vi "read max #frames.vi"(8 "error in (no error)":errorcluster, 11 "Simulated_CCD_Camera in":refnum<class "Sim_CCD.lvclass">) -> (0 "error out":errorcluster, 2 "max #pix":i64[][](array[numeric]), 3 "Simulated_CCD_Camera out":refnum<class "Sim_CCD.lvclass">)   [LabVIEW 2018, in "Sim_CCD.lvclass"]
uses:
  Sim_CCD.lvclass
  Sim_CCD.lvclass/Sim_CCD.ctl
  <vilib>/Utility/file.llb/Read Delimited Spreadsheet (I64).vi
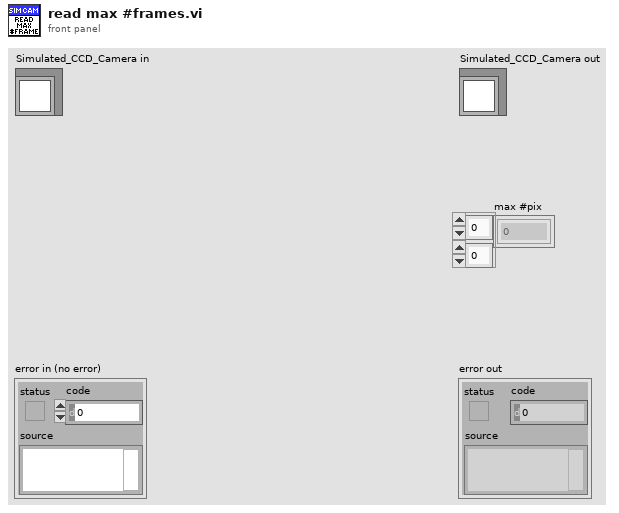
[diagram p1: front panel]
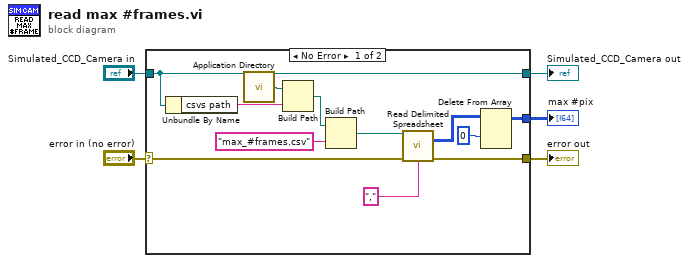
[diagram p0: block diagram]
diagram:
  n1 = case shown="No Error" "error in (no error)" {
    selector: "error in (no error)" -> [w16 w19]
    tunnel: [w15 w19] -> w4
    tunnel: [w14 w18] -> w2
    tunnel: "Simulated_CCD_Camera in" -> [w14 w18]
    tunnel: [w7 _] -> w1
    frame No Error {
      n2 = Unbundle By Name(w14) -> ("csvs path"=w9:string)
      n3 = call <vilib>:"Application Directory.vi"() -> ("Application Directory"=w13:path)
      n4 = Build Path(base path=w13, name or relative path=w9) -> (appended path=w12:path)
      n5 = Build Path(base path=w12, name or relative path="max_#frames.csv") -> (appended path=w10:path)
      n6 = call-poly <vilib>:"Read Delimited Spreadsheet.vi"("file path (dialog if empty)"=w10, "error in (no error)"=w16, "delimiter (\\t)"="," ("delimiter (\\t)")) -> ("all rows"=w8:i64[][], "error out"=w15:errorcluster)  [unwired: 7 in, 4 out]
      n7 = Delete From Array(array=w8, index (row)=0) -> (array with subset deleted=w7:i64[][])  [unwired: 2 in, 1 out]
    }
    frame Error {
    }
  }
  "error out" <- w4
  "Simulated_CCD_Camera out" <- w2
  "max #pix" <- w1
